vi "ConfigINI.vi"() -> ()   [LabVIEW 2014]
uses:
  <vilib>/Utility/config.llb/Read Key (Boolean).vi
  <vilib>/Utility/config.llb/Read Key (Double).vi
  <vilib>/Utility/config.llb/Read Key (Path).vi
  <vilib>/Utility/config.llb/NI_LVConfig.lvlib
panel:
  out "value 2":path
  out "value":dbl
  out "Boolean":bool
  in  "stop":bool
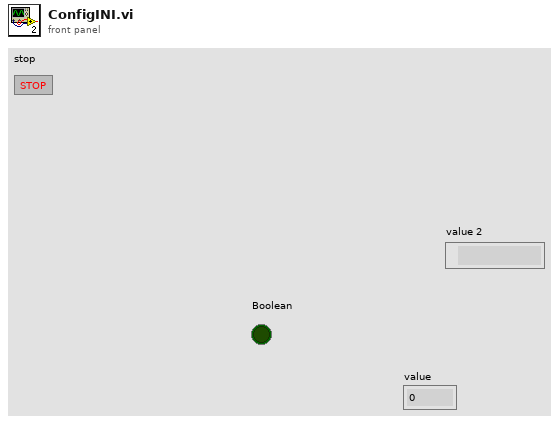
[diagram p1: front panel]
types:
  T1 = typedef "NI_LVConfig.lvlib/Config Data RefNum.ctl" = refnum<k1>
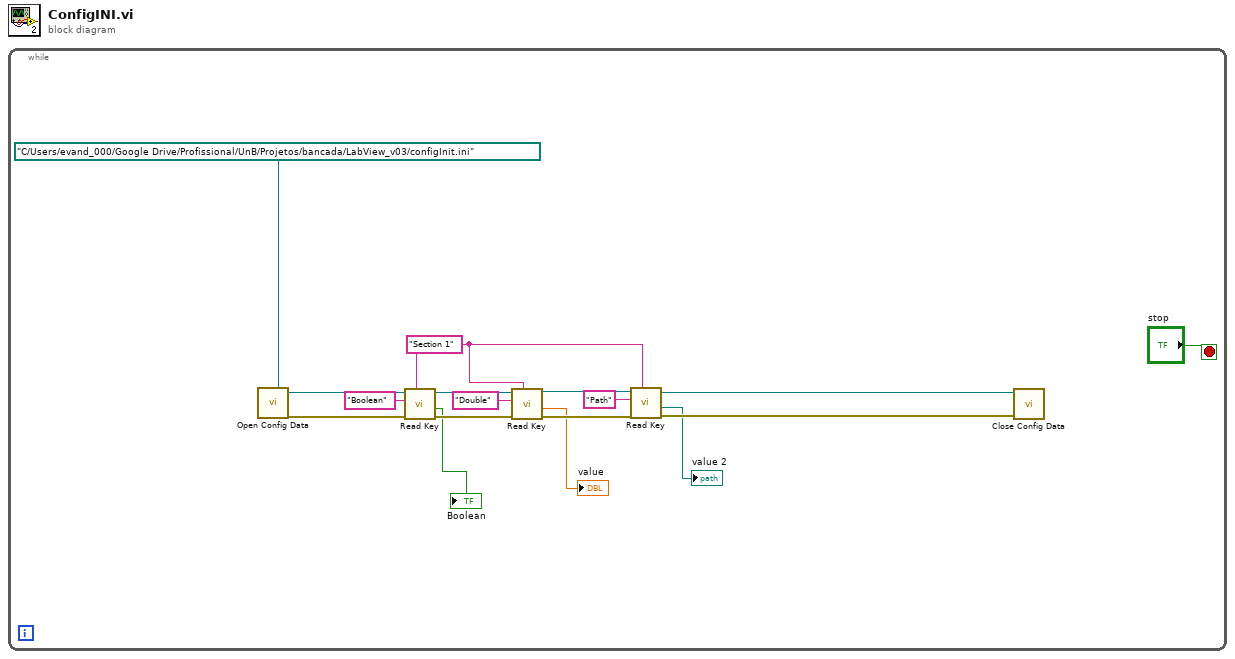
[diagram p0: block diagram]
diagram:
  n1 = while {
    stop <- "stop" stop-if-true
    w15 = "Section 1" ("section")
    n2 = call <vilib>:"Open Config Data.vi"("configuration file path"=path "C:/Users/evand_000/Google Drive/Profissional/UnB/Projetos/bancada/LabView_v03/configInit.ini") -> ("error out"=w14:errorcluster, "refnum"=w8:T1)  [unwired: 8 in, 1 out]
    n3 = call-poly <vilib>:"Read Key.vi"("section"=w15, "error in (no error)"=w14, "key"="Boolean", "refnum"=w8) -> ("error out"=w13:errorcluster, "value"=→"Boolean":bool, "refnum out"=w9:T1)  [unwired: 4 in, 1 out]
    n4 = call-poly <vilib>:"Read Key.vi"("section"=w15, "error in (no error)"=w13, "key"="Double", "refnum"=w9) -> ("error out"=w12:errorcluster, "value"=→"value":dbl, "refnum out"=w10:T1)  [unwired: 4 in, 1 out]
    n5 = call-poly <vilib>:"Read Key.vi"("section"=w15, "error in (no error)"=w12, "key"="Path", "refnum"=w10) -> ("error out"=w11:errorcluster, "value"=→"value 2":path, "refnum out"=w1:T1)  [unwired: 4 in, 1 out]
    n6 = call <vilib>:"Close Config Data.vi"("error in (no error)"=w11, "refnum"=w1) -> ()  [unwired: 8 in, 2 out]
  }
